vi "robust_create_timing_source.vi"(7 "frequency (1KHz)":enum16{"1kHz", "1MHz"}(ring), 8 "error in (no error)":errorcluster, 11 "name in":string="CEAS") -> (0 "error out":errorcluster, 3 "name out":string)   [LabVIEW 2015]
uses:
  <vilib>/Platform/TimedLoop/scheduler/LVUserAPI/_suppVIs/Create_1kHz_TSource.vi
  <vilib>/Platform/TimedLoop/scheduler/LVUserAPI/_suppVIs/Create_1MHz_TSource.vi
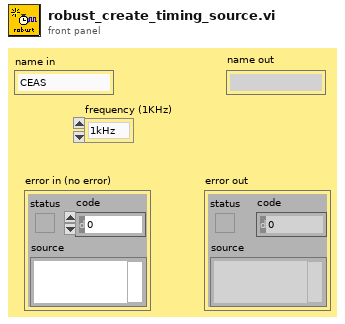
[diagram p1: front panel]
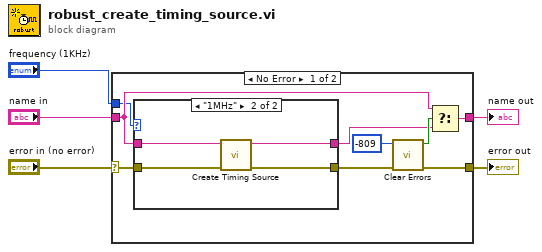
[diagram p0: block diagram]
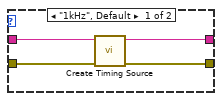
[diagram p2: hidden frame]
diagram:
  n1 = case shown="No Error" "error in (no error)" {
    selector: "error in (no error)" -> [w6 w23]
    tunnel: [w12 w23] -> w5
    tunnel: "name in" -> [w10 w24]
    tunnel: [w8 w24] -> w3
    tunnel: "frequency (1KHz)" -> [w7 _]
    frame No Error {
      n2 = case shown="\"1MHz\"" w7 {
        tunnel: [w18 w19] -> w14
        tunnel: w6 -> [w17 w20]
        tunnel: w10 -> [w16 w22]
        tunnel: [w15 w21] -> w9
        frame "1kHz", Default {
          n3 = call-poly <vilib>:"Create Timing Source.vi"("error in (no error)"=w17, "name (in)"=w16) -> ("error out"=w18:errorcluster, "name (out)"=w15:string)  [unwired: 8 in]
        }
        frame "1MHz" {
          n4 = call-poly <vilib>:"Create Timing Source.vi"("error in (no error)"=w20, "name (in)"=w22) -> ("error out"=w19:errorcluster, "name (out)"=w21:string)  [unwired: 8 in]
        }
      }
      n5 = call <vilib>:"Clear Errors.vi"("error in (no error)"=w14, "specific error code to clear (0: all)"=-809) -> ("error out"=w12:errorcluster, "specific error cleared?"=w11:bool)  [unwired: 4 in]
      n6 = Select(t=w10, s=w11, f=w9) -> (s? t:f=w8:string)
    }
    frame Error {
    }
  }
  "error out" <- w5
  "name out" <- w3
